vi "libtiff3_writeScanLine_sep_RGBm.vi"(7 "totalpages":i32, 8 "error in (no error)":errorcluster, 9 "page":u32, 10 "Data":i16[][][](array[numeric]), 11 "Handle":i32) -> (0 "error out":errorcluster, 3 "Handle out":i32)   [LabVIEW 2012]
doc: "Write a RGB page (separate color planes) using LIBTIFFwriteScanLine to a file previously open for writing"
uses:
  C:/Program Files (x86)/GnuWin32/bin/libtiff3.dll
panel:
  out "status_compression":i32
  out "status width":i32
  out "status_length":i32
  out "status_spp":i32
  out "status_bps":i32
  out "status_orientation":i32
  out "status_planarconfig":i32
  out "status_photo":i32
  out "status_writscanline R":i32
  out "status_subfile":i32
  out "status_writedir":i32
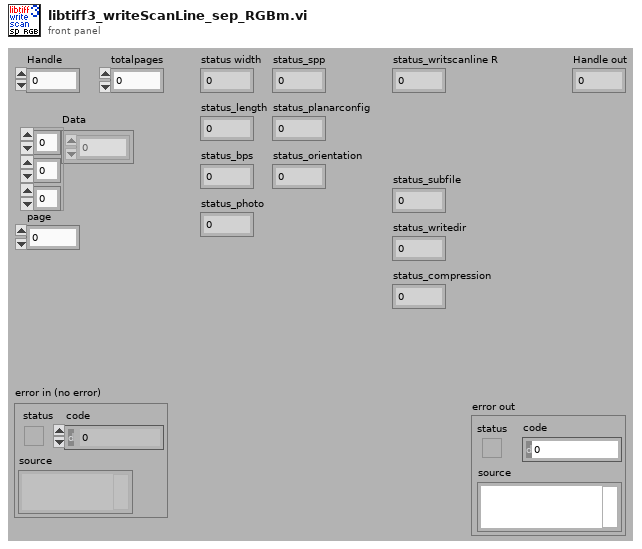
[diagram p1: front panel]
types:
  T1 = enum16{"Vertical flip", "Horizontal flip", "transpose", "rotate 90", "rotate 180", "rotate 270", "Diagonal flip"}
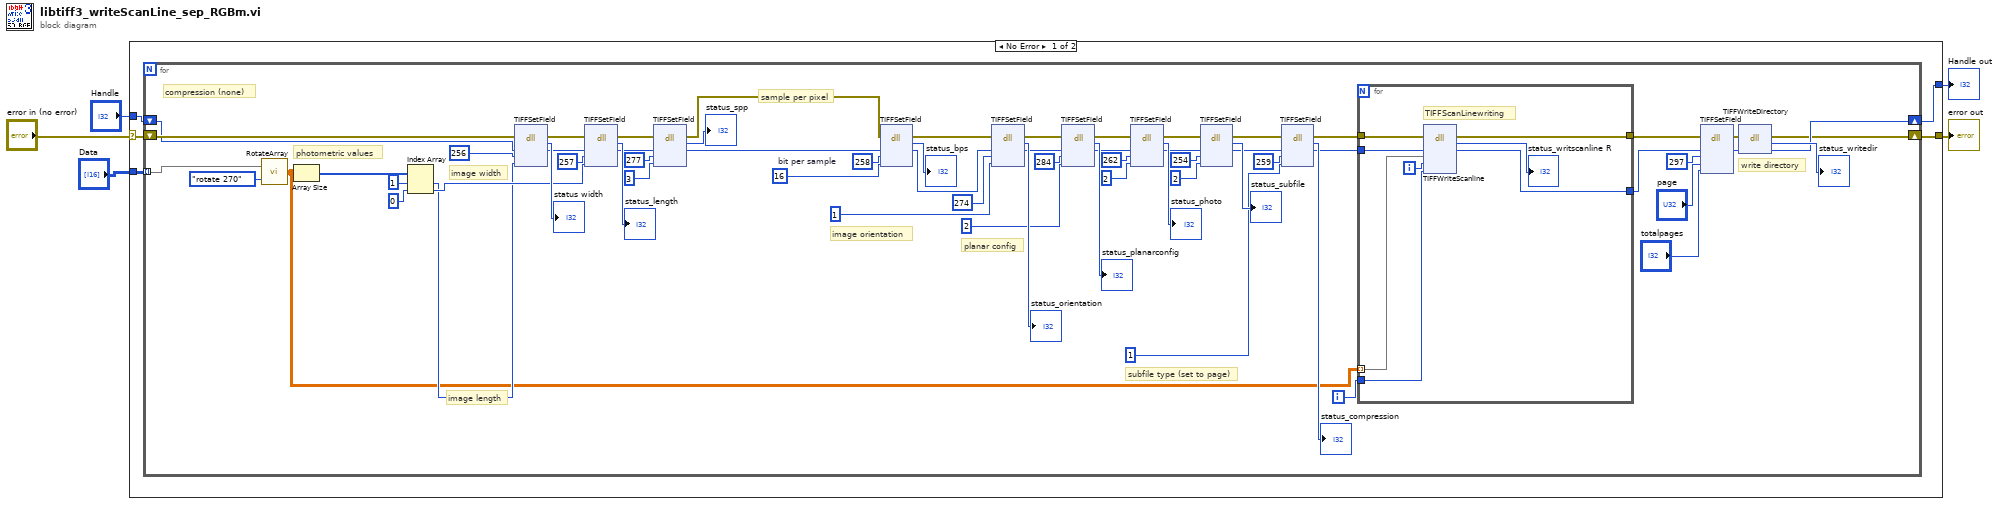
[diagram p0: block diagram]
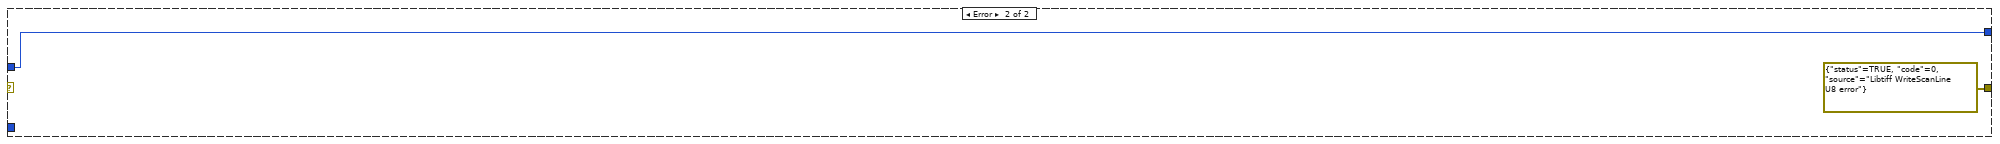
[diagram p2: hidden frame]
diagram:
  n1 = case shown="No Error" "error in (no error)" {
    selector: "error in (no error)" -> [w7 _]
    tunnel: "Handle" -> [w6 w84]
    tunnel: [w10 w84] -> w4
    tunnel: [w9 errorcluster {"status"=TRUE, "code"=0, "source"="Libtiff WriteScanLine U8 error"} ("error out")] -> w3
    tunnel: "Data" -> [w8 _]
    frame No Error {
      n2 = for {
        tunnel: w8 -> [w13] mode=indexing
        shift-right: [w29] -> w9
        shift-left: w7 -> [w17]
        shift-right: [w42] -> w10
        shift-left: w6 -> [w16]
        i -> [w15]
        w28 = u32 16  # bit per sample
        # "compression (none)"
        # "write directory"
        # "subfile type (set to page)"
        # "photometric values"
        # "planar config"
        # "image orientation"
        # "sample per pixel"
        # "image length"
        # "image width"
        n3 = call "RotateArray.vi"("Method"=T1."rotate 270", "Input"=w13) -> ("Output"=w12:dbl[][])
        n4 = Array Size(array=w12) -> (size(s)=w43:i32[])
        n5 = Index Array(array=w43, index #1=1 ("index"), index #2=0 ("index")) -> (element #1=w26:i32, element #2=w27:i32)
        n6 = dll-call lib="C:/Program Files (x86)/GnuWin32/bin/libtiff3.dll" fn="TIFFSetField"(error in=w17, "Handle"=w16, "TIFF_tag"=256, "Value"=w26) -> (error out=w37:errorcluster, →"status width":i32, "Handle"=w72:i32)  [unwired: 4 in, 1 out]
        n7 = dll-call lib="C:/Program Files (x86)/GnuWin32/bin/libtiff3.dll" fn="TIFFSetField"(error in=w37, "Handle"=w72, "TIFF_tag"=257, "value"=w27) -> (error out=w36:errorcluster, →"status_length":i32, "Handle"=w69:i32)  [unwired: 4 in, 1 out]
        n8 = dll-call lib="C:/Program Files (x86)/GnuWin32/bin/libtiff3.dll" fn="TIFFSetField"(error in=w36, "Handle"=w69, "TIFF_tag"=277, "value"=u32 3) -> (error out=w35:errorcluster, →"status_spp":i32, "Handle"=w66:i32)  [unwired: 4 in, 1 out]
        n9 = dll-call lib="C:/Program Files (x86)/GnuWin32/bin/libtiff3.dll" fn="TIFFSetField"(error in=w35, "Handle"=w66, "TIFF_tag"=258, "value"=w28) -> (error out=w34:errorcluster, →"status_bps":i32, "Handle"=w63:i32)  [unwired: 4 in, 1 out]
        n10 = dll-call lib="C:/Program Files (x86)/GnuWin32/bin/libtiff3.dll" fn="TIFFSetField"(error in=w34, "Handle"=w63, "TIFF_tag"=274, "value"=u32 1) -> (error out=w33:errorcluster, →"status_orientation":i32, "Handle"=w59:i32)  [unwired: 4 in, 1 out]
        n11 = dll-call lib="C:/Program Files (x86)/GnuWin32/bin/libtiff3.dll" fn="TIFFSetField"(error in=w33, "Handle"=w59, "TIFF_tag"=284, "value"=u32 2) -> (error out=w32:errorcluster, →"status_planarconfig":i32, "Handle"=w55:i32)  [unwired: 4 in, 1 out]
        n12 = dll-call lib="C:/Program Files (x86)/GnuWin32/bin/libtiff3.dll" fn="TIFFSetField"(error in=w32, "Handle"=w55, "TIFF_tag"=262, "value"=u32 2) -> (error out=w31:errorcluster, →"status_photo":i32, "Handle"=w50:i32)  [unwired: 4 in, 1 out]
        n13 = dll-call lib="C:/Program Files (x86)/GnuWin32/bin/libtiff3.dll" fn="TIFFSetField"(error in=w31, "Handle"=w50, "TIFF_tag"=254, "value"=u32 2) -> (error out=w30:errorcluster, →"status_subfile":i32, "Handle"=w39:i32)  [unwired: 4 in, 1 out]
        n14 = dll-call lib="C:/Program Files (x86)/GnuWin32/bin/libtiff3.dll" fn="TIFFSetField"(error in=w30, "Handle"=w39, "TIFF_tag"=259, "value"=u32 1) -> (error out=w18:errorcluster, →"status_compression":i32, "Handle"=w19:i32)  [unwired: 4 in, 1 out]
        n15 = for {
          tunnel: [w81] -> w24
          tunnel: [w76] -> w14
          tunnel: w19 -> [w79]
          tunnel: w18 -> [w80]
          tunnel: w12 -> [w77] mode=indexing
          tunnel: w15 -> [w75]
          i -> [w78]
          # "TIFFScanLinewriting"
          n16 = dll-call lib="C:/Program Files (x86)/GnuWin32/bin/libtiff3.dll" fn="TIFFWriteScanline"(error in=w80, "Handle"=w79, "buffer"=w77, "row"=w78, "sample"=w75) -> (error out=w76:errorcluster, "return type"=→"status_writscanline R":i32, "Handle"=w81:i32)  [unwired: 5 in, 1 out]
        }
        n17 = dll-call lib="C:/Program Files (x86)/GnuWin32/bin/libtiff3.dll" fn="TIFFSetField"(error in=w14, "Handle"=w24, "TIFF_tag"=297, "page"="page", "totalpages"="totalpages") -> (error out=w21:errorcluster, "Handle"=w20:i32)  [unwired: 5 in, 2 out]
        n18 = dll-call lib="C:/Program Files (x86)/GnuWin32/bin/libtiff3.dll" fn="TIFFWriteDirectory"(error in=w21, "Handle"=w20) -> (error out=w29:errorcluster, →"status_writedir":i32, "Handle"=w42:i32)  [unwired: 2 in, 1 out]
      }
    }
    frame Error {
    }
  }
  "Handle out" <- w4
  "error out" <- w3
